vi "metadata.update.description.request.vi"(8 "error in":errorcluster, 10 "Description":string, 11 "channel in":refnum<class "Channel.lvclass">) -> (0 "error out":errorcluster, 3 "JSON Payload":string)   [LabVIEW 2020, in "Nominal Client.lvclass"]
uses:
  Nominal Client/Nominal Client.lvclass
  submodules/nominal-streaming-labview-ffi/lv_src/Channel/Channel.lvclass
  submodules/nominal-streaming-labview-ffi/lv_src/Channel/Channel.lvclass/Channel.ctl
  submodules/nominal-streaming-labview-ffi/lv_src/Stream/Stream.lvclass/Stream.ctl
  3536d236-6dd3-40ff-a9be-19a538437cb9.vi
  f593ea07-b612-4092-bdd6-7231a3a1b6a9.vi
  5a4ea93c-afbb-4790-a514-34ee44610bed.vi
  submodules/nominal-streaming-labview-ffi/lv_src/Channel/name.get.vi
  submodules/nominal-streaming-labview-ffi/lv_src/Channel/stream.get.vi
  submodules/nominal-streaming-labview-ffi/lv_src/Stream/datasetRid.get.vi
  <vilib>/JDP Science/JSONtext/Variant to JSON Text.vi
  submodules/nominal-streaming-labview-ffi/lv_src/Stream/Stream.lvclass
  <vilib>/JDP Science/JSONtext/LVClass Serializer/JSONtext LVClass Serializer.lvclass
  Nominal Client/Nominal Client.lvclass/Nominal Client.ctl
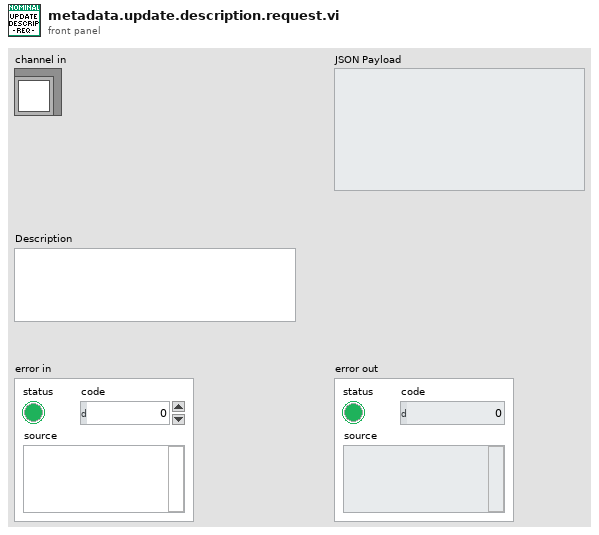
[diagram p1: front panel]
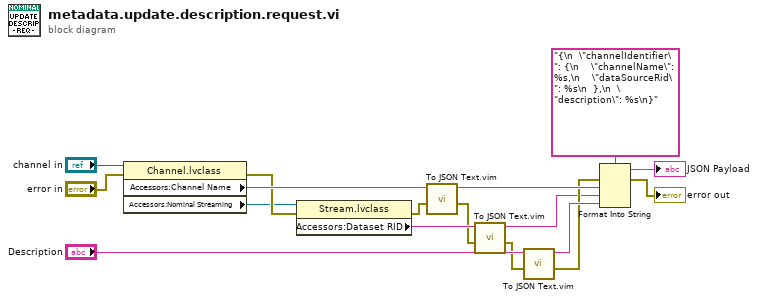
[diagram p0: block diagram]
diagram:
  n1 = property class="Channel.lvclass"(reference="channel in", error in="error in") -> (error out=w14:errorcluster, "Accessors:Channel Name"=w15:string, "Accessors:Nominal Streaming"=w8:refnum<class "Stream.lvclass">)  [unwired: 1 out]
  n2 = property class="Stream.lvclass"(reference=w8, error in=w14) -> (error out=w10:errorcluster, "Accessors:Dataset RID"=w3:string)  [unwired: 1 out]
  n3 = call "To JSON Text.vim"("error in (no error)"=w10, "Anything"=w15) -> ("error out"=w1:errorcluster, "<JSON>"=w9:string)  [unwired: 8 in]
  n4 = call "To JSON Text.vim"("error in (no error)"=w1, "Anything"=w3) -> ("error out"=w6:errorcluster, "<JSON>"=w2:string)  [unwired: 8 in]
  n5 = call "To JSON Text.vim"("error in (no error)"=w6, "Anything"="Description") -> ("error out"=w4:errorcluster, "<JSON>"=w5:string)  [unwired: 8 in]
  n6 = Format Into String(format string="{\n  \"channelIdentifier\": {\n    \"channelName\": %s,\n    \"dataSourceRid\": %s\n  },\n  \"description\": %s\n}", error in=w4, w9, w2, w5) -> (resulting string=→"JSON Payload":string, error out=→"error out":errorcluster)  [unwired: 1 in]
